vi "Acelerometro.vi"(0 "Calibrar":bool, 3 "Analog read Z":u16, 4 "Analog read Y":u16, 5 "Analog read X":u16) -> (1 "PITCH":dbl, 2 "ROLL":dbl)   [LabVIEW 2025]
doc: "VI para hacer lecturas de un acelerometro analogico tipo ADXL335 devuelve los grados en Pitch y Roll"
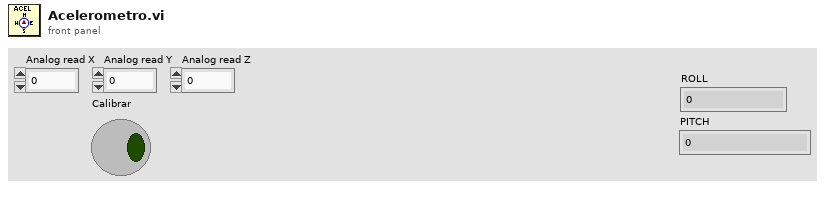
[diagram p1: front panel]
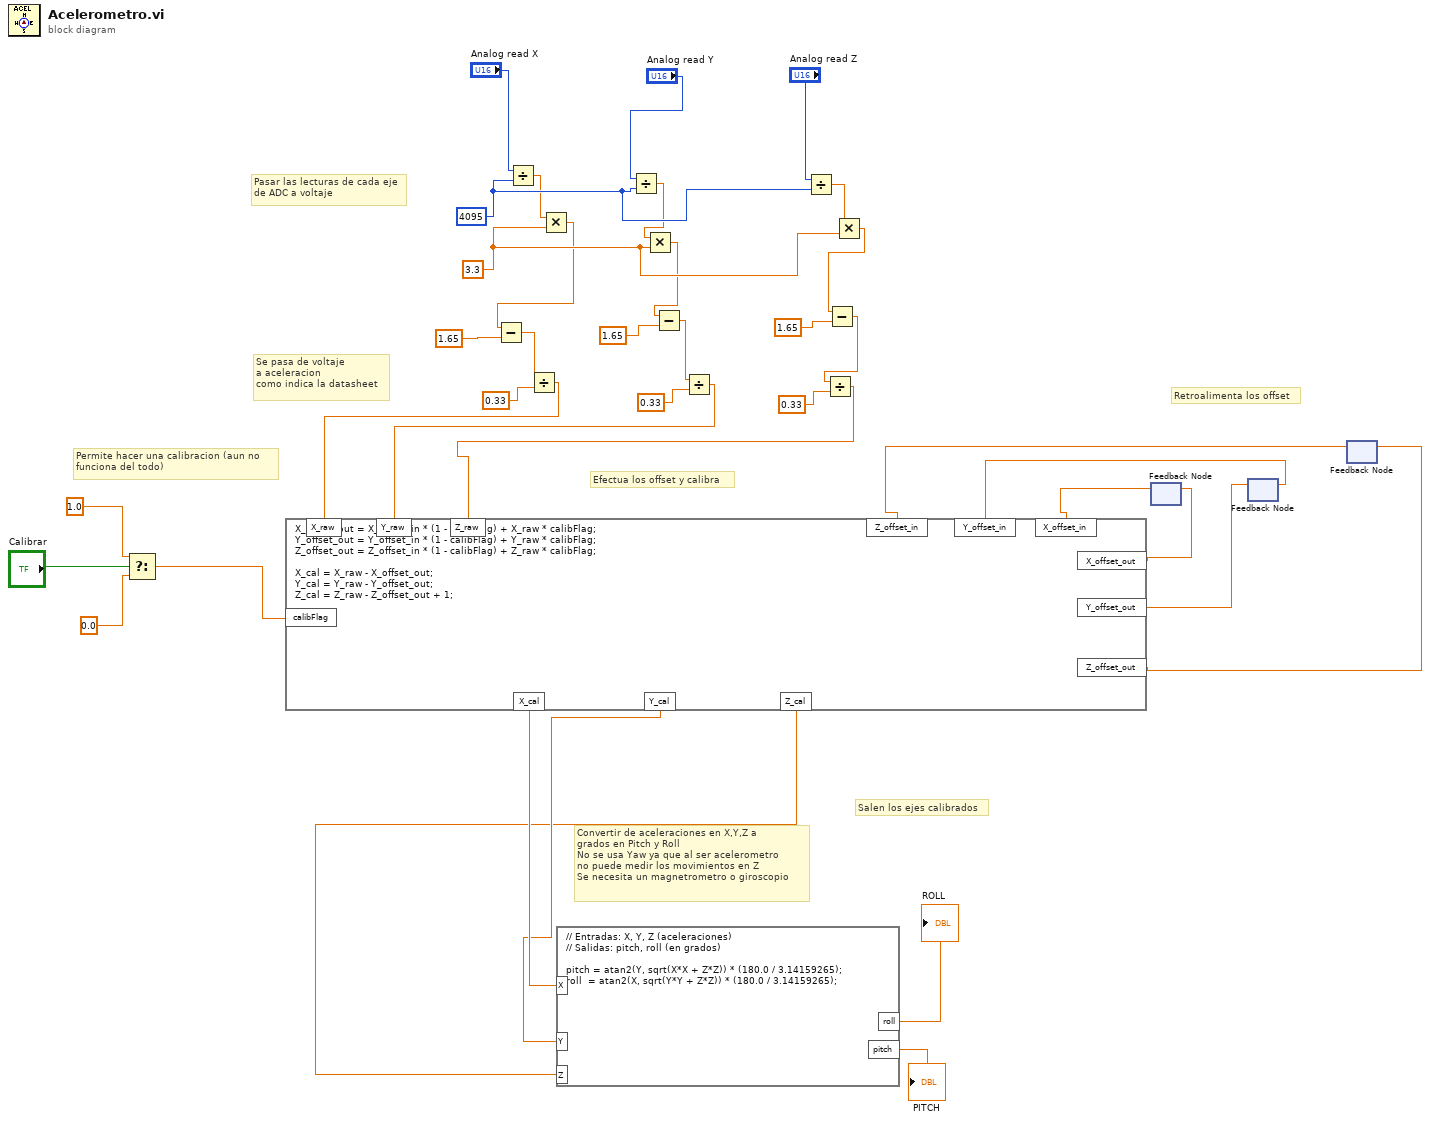
[diagram p0: block diagram]
diagram:
  w34 = 3.3
  w38 = 4095
  # "Convertir de aceleraciones en X,Y,Z a \ngrados en Pitch y Roll\nNo se usa Yaw ya que al ser acelerometro\nno puede medir los movimientos en Z \nSe necesita un magnetrometro o giroscopio"
  # "Salen los ejes calibrados"
  # "Retroalimenta los offset"
  # "Efectua los offset y calibra"
  # "Permite hacer una calibracion (aun no\nfunciona del todo)"
  # "Se pasa de voltaje \na aceleracion \ncomo indica la datasheet"
  # "Pasar las lecturas de cada eje\nde ADC a voltaje"
  n1 = Select(t=1.0, s="Calibrar", f=0.0) -> (s? t:f=w13:dbl)
  n2 = Divide(x="Analog read X", y=w38) -> (x/y=w37:dbl)
  n3 = Multiply(x=w37, y=w34) -> (x*y=w33:dbl)
  n4 = Subtract(x=w33, y=1.65) -> (x-y=w27:dbl)
  n5 = Divide(x=w27, y=0.33) -> (x/y=w12:dbl)
  n6 = Divide(x="Analog read Y", y=w38) -> (x/y=w36:dbl)
  n7 = Multiply(x=w36, y=w34) -> (x*y=w29:dbl)
  n8 = Subtract(x=w29, y=1.65) -> (x-y=w23:dbl)
  n9 = Divide(x=w23, y=0.33) -> (x/y=w11:dbl)
  n10 = Divide(x="Analog read Z", y=w38) -> (x/y=w35:dbl)
  n11 = Multiply(x=w35, y=w34) -> (x*y=w28:dbl)
  n12 = Subtract(x=w28, y=1.65) -> (x-y=w22:dbl)
  n13 = Divide(x=w22, y=0.33) -> (x/y=w10:dbl)
  n14 = feedback #1() -> (w1:dbl)  [unwired: 1 in]
  n15 = feedback #2() -> (w3:dbl)  [unwired: 1 in]
  n16 = feedback #3() -> (w5:dbl)  [unwired: 1 in]
  n17 = formula code="X_offset_out = X_offset_in * (1 - calibFlag) + X_raw * calibFlag;\nY_offset_out = Y_offset_in * (1 - calibFlag) + Y_raw * calibFlag;\nZ_offset_out = Z_offset_in * (1 - calibFlag) + Z_raw * calibFlag;\n\nX_cal = X_raw - X_offset_out;\nY_cal = Y_raw - Y_offset_out;\nZ_cal = Z_raw - Z_offset_out + 1;"("X_raw"=w12, "calibFlag"=w13, "Y_raw"=w11, "Z_raw"=w10, "X_offset_in"=w1, "Y_offset_in"=w3, "Z_offset_in"=w5) -> ("X_offset_out"=w2:dbl, "Y_offset_out"=w4:dbl, "Z_offset_out"=w6:dbl, "X_cal"=w9:dbl, "Y_cal"=w8:dbl, "Z_cal"=w7:dbl)
  n18 = formula code="// Entradas: X, Y, Z (aceleraciones)\n// Salidas: pitch, roll (en grados)\n\npitch = atan2(Y, sqrt(X*X + Z*Z)) * (180.0 / 3.14159265);\nroll  = atan2(X, sqrt(Y*Y + Z*Z)) * (180.0 / 3.14159265);"("X"=w9, "Y"=w8, "Z"=w7) -> ("pitch"=→"PITCH":dbl, "roll"=→"ROLL":dbl)
  n19 = feedback-in #1(w2) -> ()
  n20 = feedback-in #2(w4) -> ()
  n21 = feedback-in #3(w6) -> ()
